vi "Setup Connection Core.vi"(0 "Cal Standard Base in":refnum<class "Cal Standard Base.lvclass">, 5 "Path Name":string, 7 "Product Name":string, 11 "error in (no error)":errorcluster) -> (4 "Cal Standard Base out":refnum<class "Cal Standard Base.lvclass">, 15 "error out":errorcluster)   [LabVIEW 2023, in "RFFixtureCharact.Instruments.lvlib" / "Cal Standard Base.lvclass"]
uses:
  Cal Standard Base.lvclass
  Cal Standard Base.lvclass/Cal Standard Base.ctl
  Properties/Read Path Connection Map.vi
  Properties/Write Path Connection Map.vi
  <vilib>/Utility/error.llb/Trim Whitespace One-Sided.vi
  Common/RFCalAndFixtureCharact.Common.lvlib
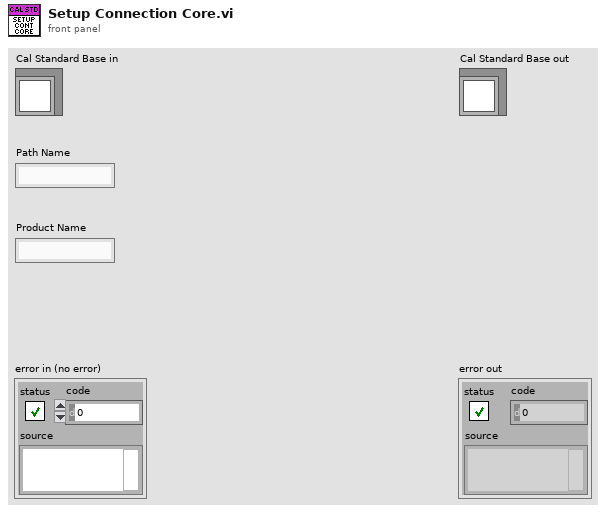
[diagram p1: front panel]
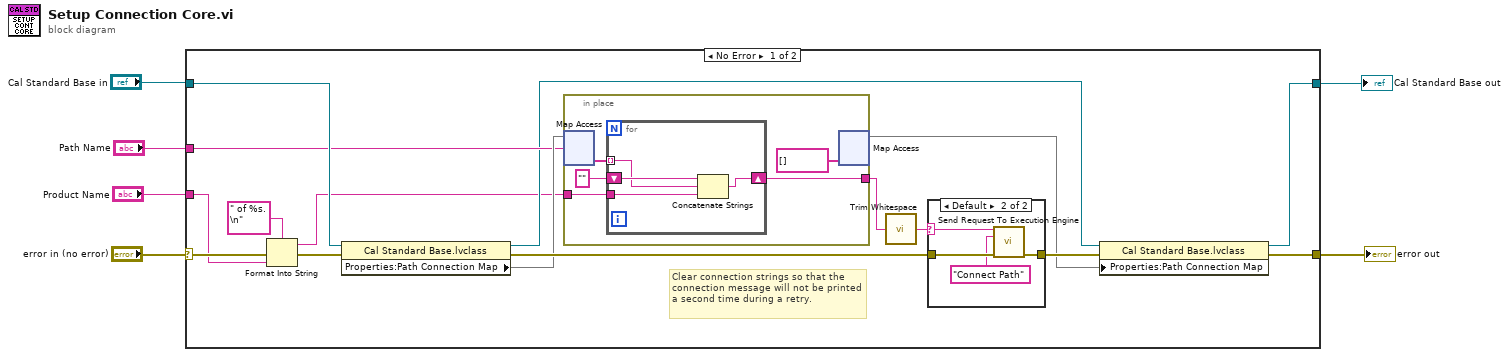
[diagram p0: block diagram]
diagram:
  n1 = case shown="No Error" "error in (no error)" {
    selector: "error in (no error)" -> [w10 w38]
    tunnel: [w17 w38] -> w2
    tunnel: [w14 w37] -> w1
    tunnel: "Cal Standard Base in" -> [w22 w37]
    tunnel: "Path Name" -> [w19 _]
    tunnel: "Product Name" -> [w8 _]
    frame No Error {
      # "Clear connection strings so that the connection message will not be printed a second time during a retry."
      n2 = Format Into String(format string=" of %s.\n" ("message"), error in=w10, w8) -> (resulting string=w7:string, error out=w9:errorcluster)  [unwired: 1 in]
      n3 = property class="Cal Standard Base.lvclass"(reference=w22, error in=w9) -> (reference out=w15:refnum<class "Cal Standard Base.lvclass">, error out=w21:errorcluster, "Properties:Path Connection Map"=w20:map{string, string[]})
      n4 = in-place {
        in-place-border: [w26] -> w13
        in-place-border: w7 -> [w23]
        n5 = in-place-map #1(w20, w19) -> (w25:string[])  [unwired: 1 in, 1 out]
        n6 = for {
          tunnel: w25 -> [w30] mode=indexing
          shift-right: [w29] -> w26
          shift-left: "" -> [w31]
          tunnel: w23 -> [w28]
          n7 = Concatenate Strings(w31, w30, w28) -> (w29:string)
        }
        n8 = in-place-map #1(string[] [] ("value")) -> (w16:map{string, string[]})  [unwired: 1 in, 2 out]
      }
      n9 = call <vilib>:"Trim Whitespace.vi"("string"=w13) -> ("trimmed string"=w12:string)  [unwired: 1 in]
      n10 = case shown="Default" w12 {
        selector: w12 -> [_ w33]
        tunnel: w21 -> [w32 w36]
        tunnel: [w32 w34] -> w18
        frame "" {
        }
        frame Default {
          n11 = call "Send Request To Execution Engine.vi"("Request Message"=w33, "Request Header"="Connect Path", "error in (no error)"=w36) -> ("error out"=w34:errorcluster)  [unwired: 11 in, 1 out]
        }
      }
      n12 = property class="Cal Standard Base.lvclass"(reference=w15, error in=w18, "Properties:Path Connection Map"=w16) -> (reference out=w14:refnum<class "Cal Standard Base.lvclass">, error out=w17:errorcluster)
    }
    frame Error {
    }
  }
  "error out" <- w2
  "Cal Standard Base out" <- w1
